vi "Video.vi"() -> ()   [LabVIEW 2011]
uses:
  <instrlib>/niHWS/nihws.llb/niHWS Open File Permissions ID.ctl
  <instrlib>/niHWS/nihws.llb/niHWS Write Analog DBL.vi
  <vilib>/vision/driver/NI_Vision_Acquisition_Software.lvlib
  <vilib>/ptbypt/NI_PtbyPt.lvlib
  C:/Program Files/National Instruments/LabVIEW 2011/resource/objmgr/imaqdx.rc
panel:
  in  "?":enum32{"Settings", "Monitor"}(tab)
  in  "Selected Path for AVI":path
  in  "Video Modes":string(combo)="1280x1024 RGB8 10.00fps"
  in  "Camera":string(combo)="uc480 Capture Device 1"
  in  "Start":bool
  in  "stop":bool
  out "Camera":T1(plugin-control)
  out "Rec Time":dbl format="%#_3g"
  in  "Display":bool=TRUE
  out "fps":dbl format="%#_2g"
  in  "Rec":bool
  # "File settings"
  # "Camera settings"
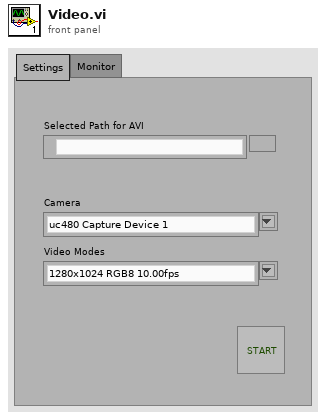
[diagram p1: front panel]
types:
  T1 = typedef "IMAQ Image.ctl" = refnum<image>
  T2 = typedef "niHWS Open File Permissions ID.ctl" = enum32{"Read Only", "Read/Write Existing", "Read/Write/Create New", "Read/Write/Create New Always"}
  T3 = cluster{"Type":u32, "Version":u32, "Flags":u32, "SerialNumberHigh":u32, "SerialNumberLow":u32, "BusType":u32, "InterfaceName":string, "VendorName":string, "ModelName":string, "CameraFileName":string, "CameraAttributeURL":string}[]
  T4 = cluster{"Type":u32, "Version":u32, "Flags":u32, "SerialNumberHigh":u32, "SerialNumberLow":u32, "BusType":u32, "InterfaceName":string, "VendorName":string, "ModelName":string, "CameraFileName":string, "CameraAttributeURL":string}
  T5 = typedef "IMAQdx.ctl" = refnum<k21>
  T6 = cluster{"Video Mode":u32, "Video Mode Name":string}[]
  T7 = typedef "AviRefnum.ctl" = refnum<k1>
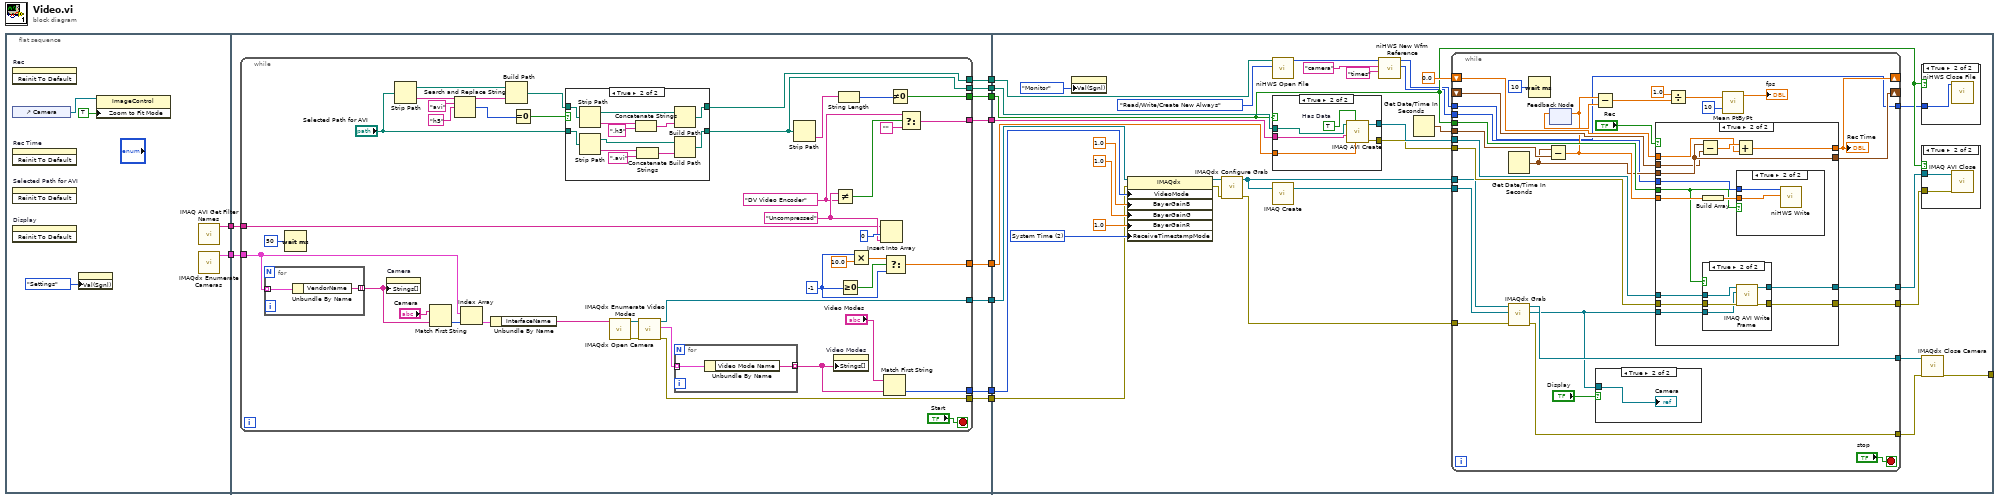
[diagram p0: block diagram]
diagram:
  n1 = flat-sequence {
    tunnel: [w12] -> w10
    tunnel: [w11] -> w9
    tunnel: [w25] -> w8
    tunnel: [w24] -> w7
    tunnel: [w23] -> w6
    tunnel: [w22] -> w5
    tunnel: [w21] -> w4
    tunnel: [w20] -> w3
    tunnel: [w19] -> w2
    tunnel: [w18] -> w1
    tunnel: w10 -> [w17]
    tunnel: w9 -> [w16]
    tunnel: w8 -> [w108]
    tunnel: w7 -> [w104]
    tunnel: w6 -> [w107]
    tunnel: w5 -> [w106]
    tunnel: w4 -> [w101]
    tunnel: w3 -> [w90]
    tunnel: w2 -> [w102]
    tunnel: w1 -> [w89]
    tunnel: [w96] -> _
    frame #0 {
      n2 = invoke on="Rec" class="Bool (strict)" method="Reinit To Default"() -> ()  [unwired: 3 in, 3 out]
      n3 = control-ref of="Camera"() -> (w15:refnum<vi>)
      n4 = invoke on="Rec Time" class="DigNum (strict)" method="Reinit To Default"() -> ()  [unwired: 3 in, 3 out]
      n5 = invoke on="Selected Path for AVI" class="Path" method="Reinit To Default"() -> ()  [unwired: 3 in, 3 out]
      n6 = invoke on="Display" class="Bool (strict)" method="Reinit To Default"() -> ()  [unwired: 3 in, 3 out]
      n7 = property class="TabCtl (strict)"("Val(Sgnl)"=enum32{"Settings", "Monitor"}."Settings" ("Value (Signaling)")) -> ()  [unwired: 2 in, 2 out]
      n8 = property on="Property Node" class="ImageControl"(reference=w15, "Zoom to Fit Mode"=TRUE) -> ()  [unwired: 1 in, 2 out]
      n9 = call "IMAQ AVI Get Filter Names"() -> ("Filter Names"=w11:string[])  [unwired: 10 in, 1 out]
      n10 = call <vilib>:"IMAQdx Enumerate Cameras.vi"() -> ("Camera Information Array"=w12:T3)  [unwired: 10 in, 1 out]
    }
    frame #1 {
      n11 = while {
        tunnel: [w50] -> w25
        tunnel: [w63] -> w24
        tunnel: [w40] -> w23
        tunnel: [w56] -> w22
        tunnel: [w31] -> w21
        tunnel: [w34] -> w20
        tunnel: [w49] -> w19
        tunnel: [w30] -> w18
        tunnel: w17 -> [w28]
        tunnel: w16 -> [w27]
        stop <- "Start" stop-if-true
        w41 = -1 ("% Quality")
        w60 = "DV Video Encoder" ("Compressor")
        w61 = "Uncompressed"
        n12 = for {
          tunnel: w28 -> [w83] mode=indexing
          tunnel: [w82] -> w55 mode=indexing
          n13 = Unbundle By Name(w83) -> ("VendorName"=w82:string)
        }
        n14 = Wait (ms)(milliseconds to wait=u32 50) -> ()  [unwired: 1 out]
        n15 = property on="Camera" class="CmbBox"("Strings[]"=w55) -> ()  [unwired: 2 in, 2 out]
        n16 = Strip Path(path="Selected Path for AVI") -> (stripped path=w48:path, name=w46:string)
        n17 = Match First String(2:w55, 3:"Camera") -> (0:w53:i32)  [unwired: 1 out]
        n18 = Search and Replace String(input string=w46, search string="avi", replace string="h5" ("replace string (\"\")")) -> (result string=w47:string, number of replacements=w37:i32)  [unwired: 5 in, 2 out]
        n19 = Index Array(array=w28, index=w53) -> (element=w52:T4)
        n20 = Unbundle By Name(w52) -> ("InterfaceName"=w51:string)
        n21 = Build Path(base path=w48, name or relative path=w47) -> (appended path=w35:path)
        n22 = Equal To 0?(x=w37) -> (x = 0?=w36:bool)
        n23 = case shown="True" w36 {
          tunnel: "Selected Path for AVI" -> [w68 w81]
          tunnel: [w68 w80] -> w31
          tunnel: w35 -> [w69 w71]
          tunnel: [w69 w70] -> w34
          frame False {
          }
          frame True {
            n24 = Strip Path(path=w71) -> (stripped path=w75:path, name=w73:string)
            n25 = Strip Path(path=w81) -> (stripped path=w79:path, name=w77:string)
            n26 = Concatenate Strings(w73, ".h5" ("search string")) -> (w72:string)
            n27 = Concatenate Strings(w77, ".avi" ("search string")) -> (w76:string)
            n28 = Build Path(base path=w75, name or relative path=w72) -> (appended path=w70:path)
            n29 = Build Path(base path=w79, name or relative path=w76) -> (appended path=w80:path)
          }
        }
        n30 = call <vilib>:"IMAQdx Open Camera.vi"("Session In"=w51) -> ("error out"=w66:errorcluster, "Session Out"=w67:T5)  [unwired: 9 in]
        n31 = call <vilib>:"IMAQdx Enumerate Video Modes.vi"("error in"=w66, "Session In"=w67) -> ("error out"=w49:errorcluster, "Video Modes"=w64:T6, "Session Out"=w50:T5)  [unwired: 6 in, 1 out]
        n32 = for {
          tunnel: w64 -> [w85] mode=indexing
          tunnel: [w84] -> w57 mode=indexing
          n33 = Unbundle By Name(w85) -> ("Video Mode Name"=w84:string)
        }
        n34 = Strip Path(path=w31) -> (name=w32:string)  [unwired: 1 out]
        n35 = Not Equal?(x=w61, y=w60) -> (x != y?=w59:bool)
        n36 = property on="Video Modes" class="CmbBox"("Strings[]"=w57) -> ()  [unwired: 2 in, 2 out]
        n37 = String Length(string=w32) -> (length=w33:i32)
        n38 = Greater Or Equal To 0?(x=w41) -> (x >= 0?=w42:bool)
        n39 = Multiply(x=w41, y=10.0) -> (x*y=w43:dbl)
        n40 = Insert Into Array(array=w27, index=0 ("Index"), new element=w61) -> ()  [unwired: 1 out]
        n41 = Match First String(2:w57, 3:"Video Modes") -> (0:w56:i32)  [unwired: 1 out]
        n42 = Select(t=w43, s=w42, f=w41) -> (s? t:f=w40:dbl)
        n43 = Not Equal To 0?(x=w33) -> (x != 0?=w30:bool)
        n44 = Select(t=w60, s=w59, f="") -> (s? t:f=w63:string)
      }
    }
    frame #2 {
      w103 = u32 2 items=["None", "Tick Count", "System Time"] ("ReceiveTimestampMode")
      n45 = property class="TabCtl (strict)"("Val(Sgnl)"=enum32{"Settings", "Monitor"}."Monitor" ("Value (Signaling)")) -> ()  [unwired: 2 in, 2 out]
      n46 = property class="IMAQdx"(reference=w108, error in=w102, "VideoMode"=w106, "BayerGainB"=1.0, "BayerGainG"=1.0, "BayerGainR"=1.0, "ReceiveTimestampMode"=w103) -> (reference out=w110:T5, error out=w109:errorcluster)
      n47 = call <vilib>:"IMAQdx Configure Grab.vi"("error in"=w109, "Session In"=w110) -> ("error out"=w114:errorcluster, "Session Out"=w105:T5)  [unwired: 8 in]
      n48 = call <instrlib>:"niHWS Open File.vi"("permissions (0:read only)"=niHWS_Open_File_Permissions_ID."Read/Write/Create New Always", "file path"=w90) -> ("file handle"=w91:u32)  [unwired: 8 in, 1 out]
      n49 = case shown="True" w89 {
        tunnel: [_ w127] -> w119
        tunnel: [_ w126] -> w116
        tunnel: w107 -> [_ w125]
        tunnel: w104 -> [_ w124]
        tunnel: w101 -> [_ w123]
        frame False {
        }
        frame True {
          w128 = TRUE  # Has Data
          n50 = call "IMAQ AVI Create"("quality"=w125, "Has Data"=w128, "Compression Filter"=w124, "AVI Path"=w123) -> ("error out"=w126:errorcluster, "Avi Refnum"=w127:T7)  [unwired: 3 in, 3 out]
        }
      }
      n51 = call "IMAQ Create"("Image Name"=w105) -> ("New Image"=w115:T1)  [unwired: 4 in, 1 out]
      n52 = call <instrlib>:"niHWS New Wfm Reference.vi"("waveform name (empty)"="times" ("group name (empty)"), "group name (empty)"="camera", "file handle in"=w91) -> ("waveform reference"=w88:u32, "file handle out"=w87:u32)  [unwired: 6 in, 1 out]
      n53 = Get Date/Time In Seconds() -> (seconds since 1Jan1904=w97:timestamp)
      n54 = while {
        tunnel: [w158] -> w118
        tunnel: [w157] -> w117
        tunnel: w119 -> [w156]
        tunnel: w116 -> [w155]
        tunnel: w115 -> [w149]
        tunnel: w105 -> [w150]
        tunnel: w114 -> [w148]
        tunnel: w97 -> [w154]
        shift-right: [w153] -> _
        shift-left: _ -> [w152]
        tunnel: w89 -> [w151]
        tunnel: [w147] -> w100
        tunnel: [w146] -> w99
        shift-right: [w144] -> _
        shift-left: 0.0 -> [w145]
        tunnel: w88 -> [w130]
        tunnel: w87 -> [w129]
        tunnel: [w129] -> w86
        stop <- "stop" stop-if-true
        n55 = Get Date/Time In Seconds() -> (seconds since 1Jan1904=w135:timestamp)
        n56 = call <vilib>:"IMAQdx Grab.vi"("error in"=w148, "Image In"=w149, "Session In"=w150) -> ("error out"=w146:errorcluster, "Image Out"=w133:T1, "Session Out"=w147:T5)  [unwired: 5 in, 1 out]
        n57 = Wait (ms)(milliseconds to wait=u32 10) -> ()  [unwired: 1 out]
        n58 = Subtract(x=w135, y=w154) -> (x-y=w136:dbl)
        n59 = feedback #1() -> (w140:dbl)  [unwired: 1 in]
        n60 = feedback-in #1(w136) -> ()
        n61 = Subtract(x=w136, y=w140) -> (x-y=w138:dbl)
        n62 = case shown="True" "Display" {
          tunnel: w133 -> [_ w184]
          frame False {
          }
          frame True {
            "Camera" <- w184
          }
        }
        n63 = case shown="True" "Rec" {
          tunnel: [w161 w176] -> w158
          tunnel: [w162 w175] -> w157
          tunnel: w156 -> [w161 w174]
          tunnel: w155 -> [w162 w173]
          tunnel: w133 -> [_ w172]
          tunnel: [w159 w165] -> w144
          tunnel: w136 -> [_ w171]
          tunnel: [w160 w168] -> w153
          tunnel: w135 -> [w160 w168]
          tunnel: w152 -> [_ w167]
          tunnel: w151 -> [_ w164]
          tunnel: w145 -> [w159 w166]
          tunnel: w130 -> [_ w163]
          frame False {
          }
          frame True {
            n64 = Subtract(x=w168, y=w167) -> (x-y=w169:dbl)
            n65 = Build Array(w171) -> (w170:dbl[])
            n66 = case shown="True" w164 {
              tunnel: [_ w181] -> w176
              tunnel: [_ w180] -> w175
              tunnel: w174 -> [_ w179]
              tunnel: w173 -> [_ w178]
              tunnel: w172 -> [_ w177]
              frame False {
              }
              frame True {
                n67 = call "IMAQ AVI Write Frame"("error in (no error)"=w178, "Image"=w177, "Avi Refnum"=w179) -> ("error out"=w180:errorcluster, "Avi Refnum (duplicate)"=w181:T7)  [unwired: 7 in]
              }
            }
            n68 = Add(x=w169, y=w166) -> (x+y=w165:dbl)
            n69 = case shown="True" w164 {
              tunnel: w170 -> [_ w183]
              tunnel: w163 -> [_ w182]
              frame False {
              }
              frame True {
                n70 = call-poly <instrlib>:"niHWS Write.vi"("data"=w183, "waveform reference in"=w182) -> ()  [unwired: 8 in, 2 out]
              }
            }
          }
        }
        "Rec Time" <- w144
        n71 = Divide(x=1.0, y=w138) -> (x/y=w137:dbl)
        n72 = call <vilib>:"Mean PtByPt.vi"("x"=w137, "sample length"=10) -> ("mean"=→"fps":dbl)  [unwired: 2 in, 1 out]
      }
      n73 = case shown="True" w89 {
        tunnel: w86 -> [_ w120]
        frame False {
        }
        frame True {
          n74 = call <instrlib>:"niHWS Close File.vi"("file handle"=w120) -> ()  [unwired: 10 in, 1 out]
        }
      }
      n75 = case shown="True" w89 {
        tunnel: w118 -> [_ w122]
        tunnel: w117 -> [_ w121]
        frame False {
        }
        frame True {
          n76 = call "IMAQ AVI Close"("error in (no error)"=w121, "Avi Refnum"=w122) -> ()  [unwired: 9 in, 1 out]
        }
      }
      n77 = call <vilib>:"IMAQdx Close Camera.vi"("error in"=w99, "Session In"=w100) -> ("error out"=w96:errorcluster)  [unwired: 9 in]
    }
  }
